vi "AO Write.vi"   [LabVIEW 2009]
doc: "Writes data into the buffer for a buffered analog output operation."
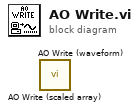
[diagram p0: block diagram]
diagram:
  n1 = call "AO Write (scaled array).vi"() -> ()  [unwired: 11 in, 5 out]
  n2 = call "AO Write (waveform).vi"() -> ()  [unwired: 11 in, 5 out]
